vi "convert result indicies to typedef data.vi"(11 "Result Indicies":i32[](array[numeric])) -> (3 "Results from processing":T1)   [LabVIEW 2013, in "fixed channel tag bus module.lvclass"]
uses:
  fixed channel tag bus module.lvclass
  results.ctl
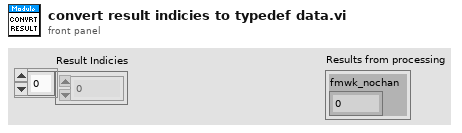
[diagram p1: front panel]
types:
  T1 = typedef "fixed channel tag bus module.lvclass/results.ctl" = cluster{"fmwk_nochan":i32}
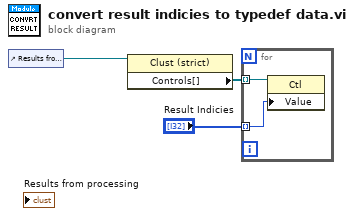
[diagram p0: block diagram]
diagram:
  n1 = control-ref of="Results from processing"() -> (w1:refnum<vi>)
  n2 = property class="Clust (strict)"(reference=w1) -> ("Controls[]"=w3:refnum<vi>[])  [unwired: 1 in, 2 out]
  n3 = for {
    tunnel: w3 -> [w5] mode=indexing
    tunnel: "Result Indicies" -> [w4] mode=indexing
    n4 = property class="Ctl"(reference=w5, "Value"=w4) -> ()  [unwired: 1 in, 2 out]
  }
